vi "RT Driver VI.vi"(7 "Operation":T1, 11 "Device Reference in":T2 format="%.0x") -> (0 "Error Code":i32)   [LabVIEW 2023, in "Ballard ARINC 429 Engine.lvlib" / "Custom Device.lvlib"]
uses:
  Custom Device.lvlib
  <vilib>/NI VeriStand/Custom Device API/Custom Device API.lvlib
  <vilib>/NI VeriStand/Custom Device Tools/Custom Device Utility Library/Custom Device Utility Library.lvlib
  <vilib>/NI VeriStand/Custom Device API/Data Reference.ctl
  <vilib>/NI VeriStand/Custom Device API/Block Data Reference.ctl
  Inline Execution Unit Runtime Information.ctl
  <vilib>/NI/NIVS Inline Async API/_VS Inline Async API/VS Inline Async API/VS Inline Async API.lvclass
  RTStateVariables.ctl
  Asynchronous Execution Unit Runtime Information.ctl
  Interfaces/Execution Unit/Execution Unit.lvclass
  Scripting/Ballard/Constants.vi
  Scripting/Ballard/Ballard ARINC 429 Scripting.lvlib
  Inline Execution Unit Compiled Information.ctl
  Asynchronous Execution Unit Compiled Information.ctl
  Compiled.Settings.ctl
  <vilib>/NI VeriStand/Custom Device API/Get Item Property (Variant).vi
  Interfaces/Shared Resources/Shared Resources.lvclass
  <vilib>/NI VeriStand/Custom Device API/Custom Device Item Ref.ctl
  <vilib>/NI VeriStand/Custom Device API/Hardware Interface Driver VI Operation.ctl
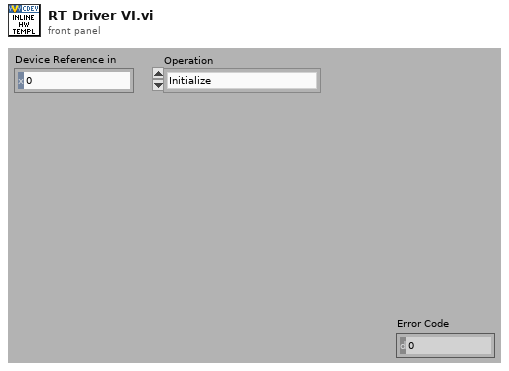
[diagram p1: front panel]
types:
  T1 = typedef "Custom Device API.lvlib/Hardware Interface Driver VI Operation.ctl" = enum16{"Initialize", "Start", "Read Data from HW", "Write Data to HW", "Close"}
  T2 = typedef "Custom Device API.lvlib/Custom Device Item Ref.ctl" = u64
  T3 = typedef "Ballard ARINC 429 Engine.lvlib/Custom Device.lvlib/RTStateVariables.ctl" = cluster{"Async":refnum<class "VS Inline Async API.lvclass">, "Inline Execution Units":T4[], "Asynchronous Execution Units":T7[], "shared resources":refnum<class "Shared Resources.lvclass">}
  T4 = typedef "Ballard ARINC 429 Engine.lvlib/Custom Device.lvlib/Inline Execution Unit Runtime Information.ctl" = cluster{"Execution Unit":refnum<class "Execution Unit.lvclass">, "Incoming Buffer":dbl[], "Outgoing Buffer":dbl[], "Incoming Data References":T5[], "Outgoing Data References":T6[]}
  T5 = typedef "Custom Device API.lvlib/Data Reference.ctl" = i32
  T6 = typedef "Custom Device API.lvlib/Block Data Reference.ctl" = cluster{"Data Reference":T5, "Offset":u64, "Length":u64}
  T7 = typedef "Ballard ARINC 429 Engine.lvlib/Custom Device.lvlib/Asynchronous Execution Unit Runtime Information.ctl" = cluster{"Execution Unit":refnum<class "Execution Unit.lvclass">, "Incoming Channel Group Name":string, "Outgoing Channel Group Name":string, "ReadWrite Channel Group Name":string}
  T8 = typedef "Ballard ARINC 429 Engine.lvlib/Custom Device.lvlib/Compiled.Settings.ctl" = cluster{"Name":string, "Inline Execution Unit Compiled Information":T9[], "Asynchronous Execution Unit Compiled Information":cluster{"Grouped Asynchronous Execution Unit Compiled Information":T10[]}[], "flattened shared resources":string}
  T9 = typedef "Ballard ARINC 429 Engine.lvlib/Custom Device.lvlib/Inline Execution Unit Compiled Information.ctl" = cluster{"Flattened Execution Unit":string, "Incoming Buffer":dbl[], "Outgoing Buffer":dbl[], "Incoming Data References":T5[], "Outgoing Data References":T6[]}
  T10 = typedef "Ballard ARINC 429 Engine.lvlib/Custom Device.lvlib/Asynchronous Execution Unit Compiled Information.ctl" = cluster{"Flattened Execution Unit":string, "Incoming Channel Group Name":string, "Outgoing Channel Group Name":string, "ReadWrite Channel Group Name":string}
  T11 = typedef "Ballard ARINC 429 Engine.lvlib/Custom Device.lvlib/RTStateVariables.ctl" = cluster{"Async":refnum<class "VS Inline Async API.lvclass">, "Inline Execution Units":T4[], "Asynchronous Execution Units":cluster{"Grouped Asynchronous Execution Units":T7[]}[], "shared resources":refnum<class "Shared Resources.lvclass">}
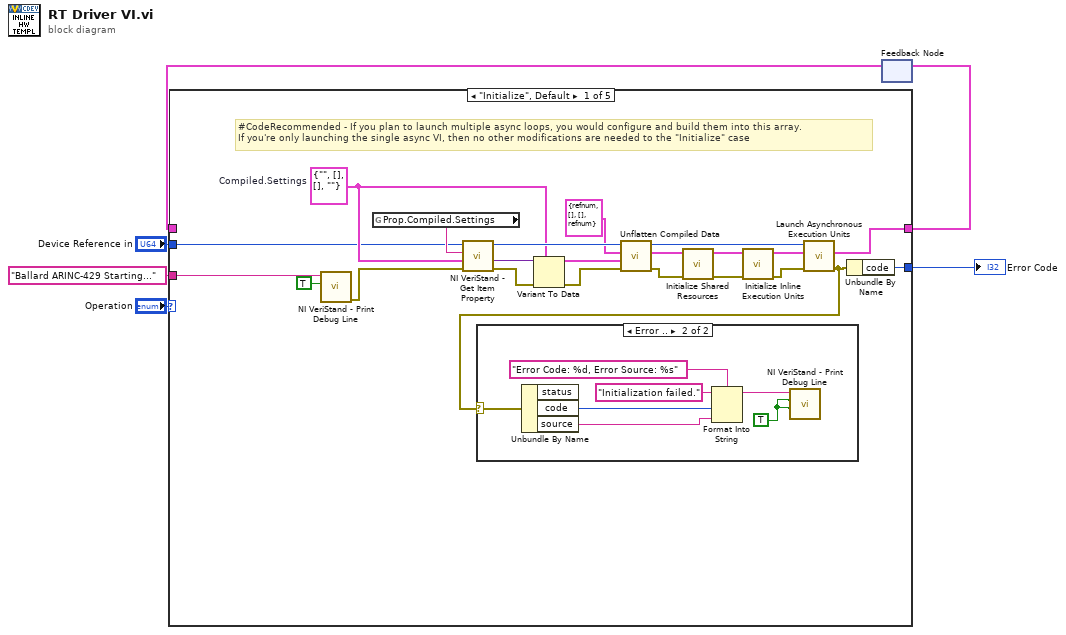
[diagram p0: block diagram]
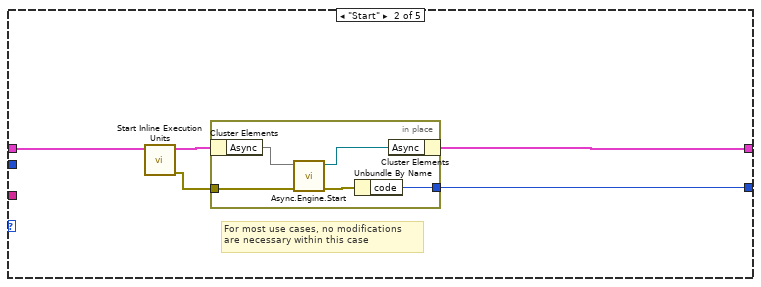
[diagram p3: hidden frame]
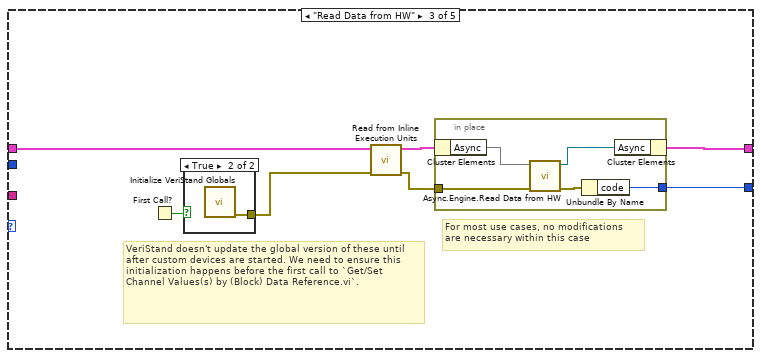
[diagram p4: hidden frame]
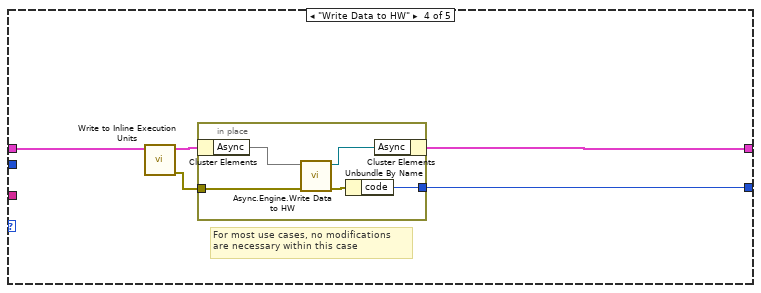
[diagram p6: hidden frame]
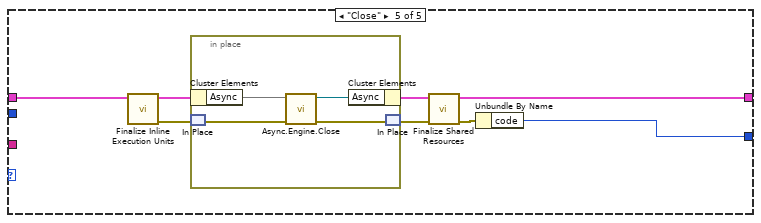
[diagram p7: hidden frame]
diagram:
  n1 = feedback #1() -> (w4:T3)  [unwired: 1 out]
  n2 = case shown="\"Initialize\", Default" "Operation" {
    tunnel: [w27 w39 w51 w62 w70] -> w5
    tunnel: w4 -> [_ w40 w50 w61 w76]
    tunnel: "Device Reference in" -> [w15 _ _ _ _]
    tunnel: [w28 w38 w52 w63 w74] -> w2
    tunnel: "Ballard ARINC-429 Starting..." ("Message") -> [w26 _ _ _ _]
    frame "Initialize", Default {
      w17 = T8 {"Name"="", "Inline Execution Unit Compiled Information"=[], "Asynchronous Execution Unit Compiled Information"=[], "flattened shared resources"=""}  # Compiled.Settings
      # "#CodeRecommended - If you plan to launch multiple async loops, you would configure and build them into this array. \nIf you're only launching the single async VI, then no other modifications are needed to the \"Initialize\" case"
      n3 = call <vilib>:"NI VeriStand - Print Debug Line.vi"("Add to log file? (F)"=TRUE, "Message"=w26) -> ("error out"=w12:errorcluster)  [unwired: 9 in]
      n4 = global read "Constants.vi" "Prop.Compiled.Settings"() -> (w16:string)
      n5 = call-poly <vilib>:"NI VeriStand - Get Item Property.vi"("error in (no error)"=w12, "Default Value"=w17, "Property Name"=w16, "Item Ref in"=w15) -> ("error out"=w21:errorcluster, "Value"=w23:variant, "Item Ref out"=w22:T2)  [unwired: 4 in, 1 out]
      n6 = Variant To Data(error in=w21, type=w17, Variant=w23) -> (data=w18:T8, error out=w10:errorcluster)
      n7 = call "Unflatten Compiled Data.vi"("error in"=w10, "Compiled.Settings"=w18, "RTStateVariables in"=T3 {"Async"=refnum, "Inline Execution Units"=[], "Asynchronous Execution Units"=[], "shared resources"=refnum} ("RTStateVariables"), "Item Ref in"=w22) -> ("error out"=w11:errorcluster, "RTStateVariables out"=w14:T11, "Item Ref out"=w24:T2)  [unwired: 5 in]
      n8 = call "Initialize Shared Resources.vi"("error in"=w11, "RTStateVariables in"=w14) -> ("error out"=w9:errorcluster, "RTStateVariables out"=w13:T3)  [unwired: 6 in]
      n9 = call "Initialize Inline Execution Units.vi"("error in"=w9, "RTStateVariables in"=w13) -> ("error out"=w8:errorcluster, "RTStateVariables out"=w25:T3)  [unwired: 8 in]
      n10 = call "Launch Asynchronous Execution Units.vi"("error in"=w8, "RTStateVariables in"=w25, "Device Ref in"=w24) -> ("error out"=w7:errorcluster, "RTStateVariables out"=w27:T11)  [unwired: 6 in, 1 out]
      n11 = case shown="Error .." w7 {
        selector: w7 -> [_ w35]
        frame No Error {
        }
        frame Error {
          w29 = TRUE ("Add to log file? (F)")
          n12 = Unbundle By Name(w35) -> ("code"=w32:i32, "source"=w31:string)  [unwired: 1 out]
          n13 = Format Into String(format string="Error Code: %d, Error Source: %s", initial string="Initialization failed.", w32, w31) -> (resulting string=w30:string)  [unwired: 1 in, 1 out]
          n14 = call <vilib>:"NI VeriStand - Print Debug Line.vi"("Append newline? (T)"=w29, "Add to log file? (F)"=w29, "Message"=w30) -> ()  [unwired: 8 in, 1 out]
        }
      }
      n15 = Unbundle By Name(w7) -> ("code"=w28:i32)
    }
    frame "Start" {
      # "For most use cases, no modifications \nare necessary within this case"
      n16 = call "Start Inline Execution Units.vi"("RTStateVariables in"=w40) -> ("error out"=w36:errorcluster, "RTStateVariables out"=w37:T3)  [unwired: 9 in]
      n17 = in-place {
        in-place-border: [w42] -> w38
        in-place-border: w36 -> [w41]
        n18 = in-place-cluster #2(w37) -> ("Async"=w45)
        n19 = call <vilib>:"Async.Engine.Start.vi"("error in (no error)"=w41, "VS Inline Async API in"=w45) -> ("error out"=w43:errorcluster, "VS Inline Async API out"=w44:refnum<class "VS Inline Async API.lvclass">)  [unwired: 8 in]
        n20 = Unbundle By Name(w43) -> ("code"=w42:i32)
        n21 = in-place-cluster #2("Async"=w44) -> (w39:cluster{})
      }
    }
    frame "Read Data from HW" {
      # "VeriStand doesn't update the global version of these until after custom devices are started. We need to ensure this initialization happens before the first call to `Get/Set Channel Values(s) by (Block) Data Reference.vi`."
      # "For most use cases, no modifications \nare necessary within this case"
      n22 = First Call?() -> (First Call?: T/F=w47:bool)
      n23 = case shown="True" w47 {
        tunnel: [_ w53] -> w46
        frame False {
        }
        frame True {
          n24 = call "Initialize VeriStand Globals.vi"() -> ("error out"=w53:errorcluster)  [unwired: 11 in]
        }
      }
      n25 = call "Read from Inline Execution Units.vi"("error in (no error)"=w46, "RTStateVariables in"=w50) -> ("error out"=w48:errorcluster, "RTStateVariables out"=w49:T3)  [unwired: 8 in]
      n26 = in-place {
        in-place-border: [w56] -> w52
        in-place-border: w48 -> [w54]
        n27 = in-place-cluster #3(w49) -> ("Async"=w58)
        n28 = call <vilib>:"Async.Engine.Read Data from HW.vi"("error in"=w54, "Async in"=w58) -> ("error out"=w55:errorcluster, "Async out"=w57:refnum<class "VS Inline Async API.lvclass">)  [unwired: 8 in]
        n29 = Unbundle By Name(w55) -> ("code"=w56:i32)
        n30 = in-place-cluster #3("Async"=w57) -> (w51:cluster{})
      }
    }
    frame "Write Data to HW" {
      # "For most use cases, no modifications \nare necessary within this case"
      n31 = call "Write to Inline Execution Units.vi"("RTStateVariables in"=w61) -> ("error out"=w59:errorcluster, "RTStateVariables out"=w60:T3)  [unwired: 9 in]
      n32 = in-place {
        in-place-border: [w68] -> w63
        in-place-border: w59 -> [w64]
        n33 = in-place-cluster #4(w60) -> ("Async"=w66)
        n34 = call <vilib>:"Async.Engine.Write Data to HW.vi"("error in (no error)"=w64, "VS Inline Async API in"=w66) -> ("error out"=w67:errorcluster, "VS Inline Async API out"=w65:refnum<class "VS Inline Async API.lvclass">)  [unwired: 8 in]
        n35 = Unbundle By Name(w67) -> ("code"=w68:i32)
        n36 = in-place-cluster #4("Async"=w65) -> (w62:cluster{})
      }
    }
    frame "Close" {
      n37 = call "Finalize Inline Execution Units.vi"("RTStateVariables in"=w76) -> ("error out"=w73:errorcluster, "RTStateVariables out"=w75:T3)  [unwired: 9 in]
      n38 = in-place {
        n39 = in-place-cluster #5(w75) -> ("Async"=w80)
        n40 = in-place-match #6(w73) -> (w78:errorcluster)
        n41 = call <vilib>:"Async.Engine.Close.vi"("error in (no error)"=w78, "Async in"=w80) -> ("error out"=w77:errorcluster, "Async out"=w79:refnum<class "VS Inline Async API.lvclass">)  [unwired: 8 in]
        n42 = in-place-cluster #5("Async"=w79) -> (w71:cluster{})
        n43 = in-place-match #6(w77) -> (w72:errorcluster)
      }
      n44 = call "Finalize Shared Resources.vi"("error in"=w72, "RTStateVariables in"=w71) -> ("error out"=w69:errorcluster, "RTStateVariables out"=w70:T3)  [unwired: 8 in]
      n45 = Unbundle By Name(w69) -> ("code"=w74:i32)
    }
  }
  "Error Code" <- w2
  n46 = feedback-in #1(w5) -> ()
